vi "writeChannelSubVI.vi"(1 "data":bool, 2 "lines":tag, 3 "error in":errorcluster, 4 "name to assign":string) -> (0 "error out":errorcluster)   [LabVIEW 2015]
doc: "Write Digital Output Port 1 Line\n=====================\n\nInput\n------\nname to assign : Name to Channel\nlines : Device's Port Line\ndata : Boolean type\n\nOutput\n--------\nerror out: Error"
uses:
  <vilib>/DAQmx/write.llb/DAQmx Write (Digital Bool 1Line 1Point).vi
  <vilib>/DAQmx/create/channels.llb/DAQmx Create Channel (DO-Digital Output).vi
  <vilib>/DAQmx/miscellaneous.llb/DAQmx Fill In Error Info.vi
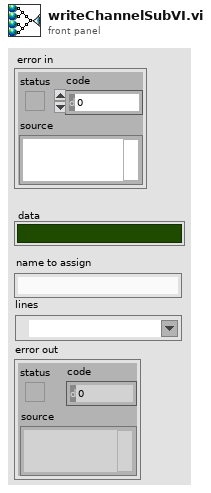
[diagram p1: front panel]
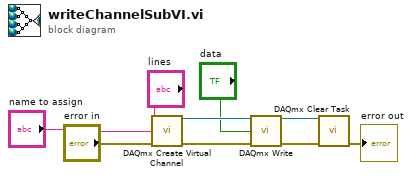
[diagram p0: block diagram]
diagram:
  n1 = call-poly <vilib>:"DAQmx Create Virtual Channel.vi"("lines"="lines", "name to assign"="name to assign", "error in"="error in") -> ("task out"=w7:refnum<k21>, "error out"=w6:errorcluster)  [unwired: 11 in]
  n2 = call-poly <vilib>:"DAQmx Write.vi"("task/channels in"=w7, "data"="data", "error in"=w6) -> ("task out"=w8:refnum<k21>, "error out"=w9:errorcluster)  [unwired: 10 in, 1 out]
  n3 = call <vilib>:"DAQmx Clear Task.vi"("task in"=w8, "error in"=w9) -> ("error out"=→"error out":errorcluster)  [unwired: 13 in]
